vi "measure_j-v.vi"(4 "Skip pixel?":bool, 5 "Date array":string[](array[string]), 6 "Scan settings":T1={"J-V scan"=TRUE, "J-t scan"=FALSE, "Min voltage (V)"=0.0, "Max voltage (V)"=1.4, "Step (V)"=0.01, "Measurement delay (ms)"=10.0, "1st scan FB-SC"=TRUE, "Inverted structure"=FALSE, "Stabilisation time (s)"=0.0, "Stabilisation mode"=0, "Stabilisation value (V or A) "=0.0, "Step time (s)"=1.0, "Integration time"=0, "Repeat light scans"=FALSE, "Stabilisation in the dark?"=FALSE, "J-t Min (V)"=0.0, "J-t Max (V)"=1.4, "J-t Step (V)"=0.01, "Max. power stabilisation"=FALSE, "J-t 1st scan FB-SC"=TRUE, "J-t Inverted structure"=FALSE, "Max power tracking"=FALSE, "Vmp (V)"=0.7, "Total stabilisation time (s)"=100.0, "J-t best pixel only"=0, "Max power best pixel only"=0, "Vmp from J-V scan"=FALSE, "No. of repeat scans"=2.0, "Only repeat for best pixel"=0, "Stabilisation time step (s)"=1.0, "Illumination conditions"=2, "Scan rate min (V/s)"=0.1, "Scan rate max (V/s)"=1.0, "No. of scan rate steps"=1.0, "Scan rate voltage step priority"=FALSE, "Scan rate measurement delay priority"=FALSE, "J-t Illumination conditions"=0, "Max P stab. Specific voltage"=FALSE} {"J-t Illumination conditions" items=["Light only", "Dark only", "Light then dark", "Dark then light"]; "No. of scan rate steps" min=1.0 step=1.0; "Illumination conditions" items=["Light only", "Dark only", "Light then dark", "Dark then light", "Light then dark then light", "Dark then light then dark"]; "Only repeat for best pixel" items=["only for best pixel", "for best 2 pixels", "for best 3 pixels", "for best 4 pixels", "for best 5 pixels", "for best 6 pixels", "for best 7 pixels", "for all pixels"]; "No. of repeat scans" min=1.0 step=1.0; "Max power best pixel only" items=["only the best pixel", "the best 2 pixels", "the best 3 pixels", "the best 4 pixels", "the best 5 pixels", "the best 6 pixels", "the best 7 pixels", "all pixels"]; "J-t best pixel only" items=["only the best pixel", "the best 2 pixels", "the best 3 pixels", "the best 4 pixels", "the best 5 pixels", "the best 6 pixels", "the best 7 pixels", "all pixels"]; "Integration time" items=["Fast", "Normal", "High Accuracy"]; "Stabilisation mode" items=["V", "I"]; "Measurement delay (ms)" min=10.0}, 7 "Cell details cluster":T3={"Cell Position"=16, "Cell Label"="", "Pixel to measure"=0, "Area (cm^2)"=0.126, "Variable"="", "Variable value"="", "Scan settings in queue"=0, "Light or dark"="", "Measurement type"=""} {"Pixel to measure" items=["All", "1", "2", "3", "4", "5", "6", "7", "8"]}, 8 "Intensity (no. of suns)":string, 9 "Scan rate (V/s)":dbl, 10 "Experiment Title":string, 11 "User Name":string) -> (0 "Log Table":string[][](table), 2 "File path for master log":path, 3 "JV Curve":cluster{"Y":dbl[], "Y":dbl[]}[](graph))   [LabVIEW 2016]
uses:
  TypeDefs/scan_settings.ctl
  TypeDefs/Settings Boolean.ctl
  TypeDefs/nplc_for_j-v_scan.ctl
  <instrlib>/Keithley 24XX/Public/Data/Read (Single Point).vi
  <instrlib>/Keithley 24XX/Keithley 24XX.lvlib
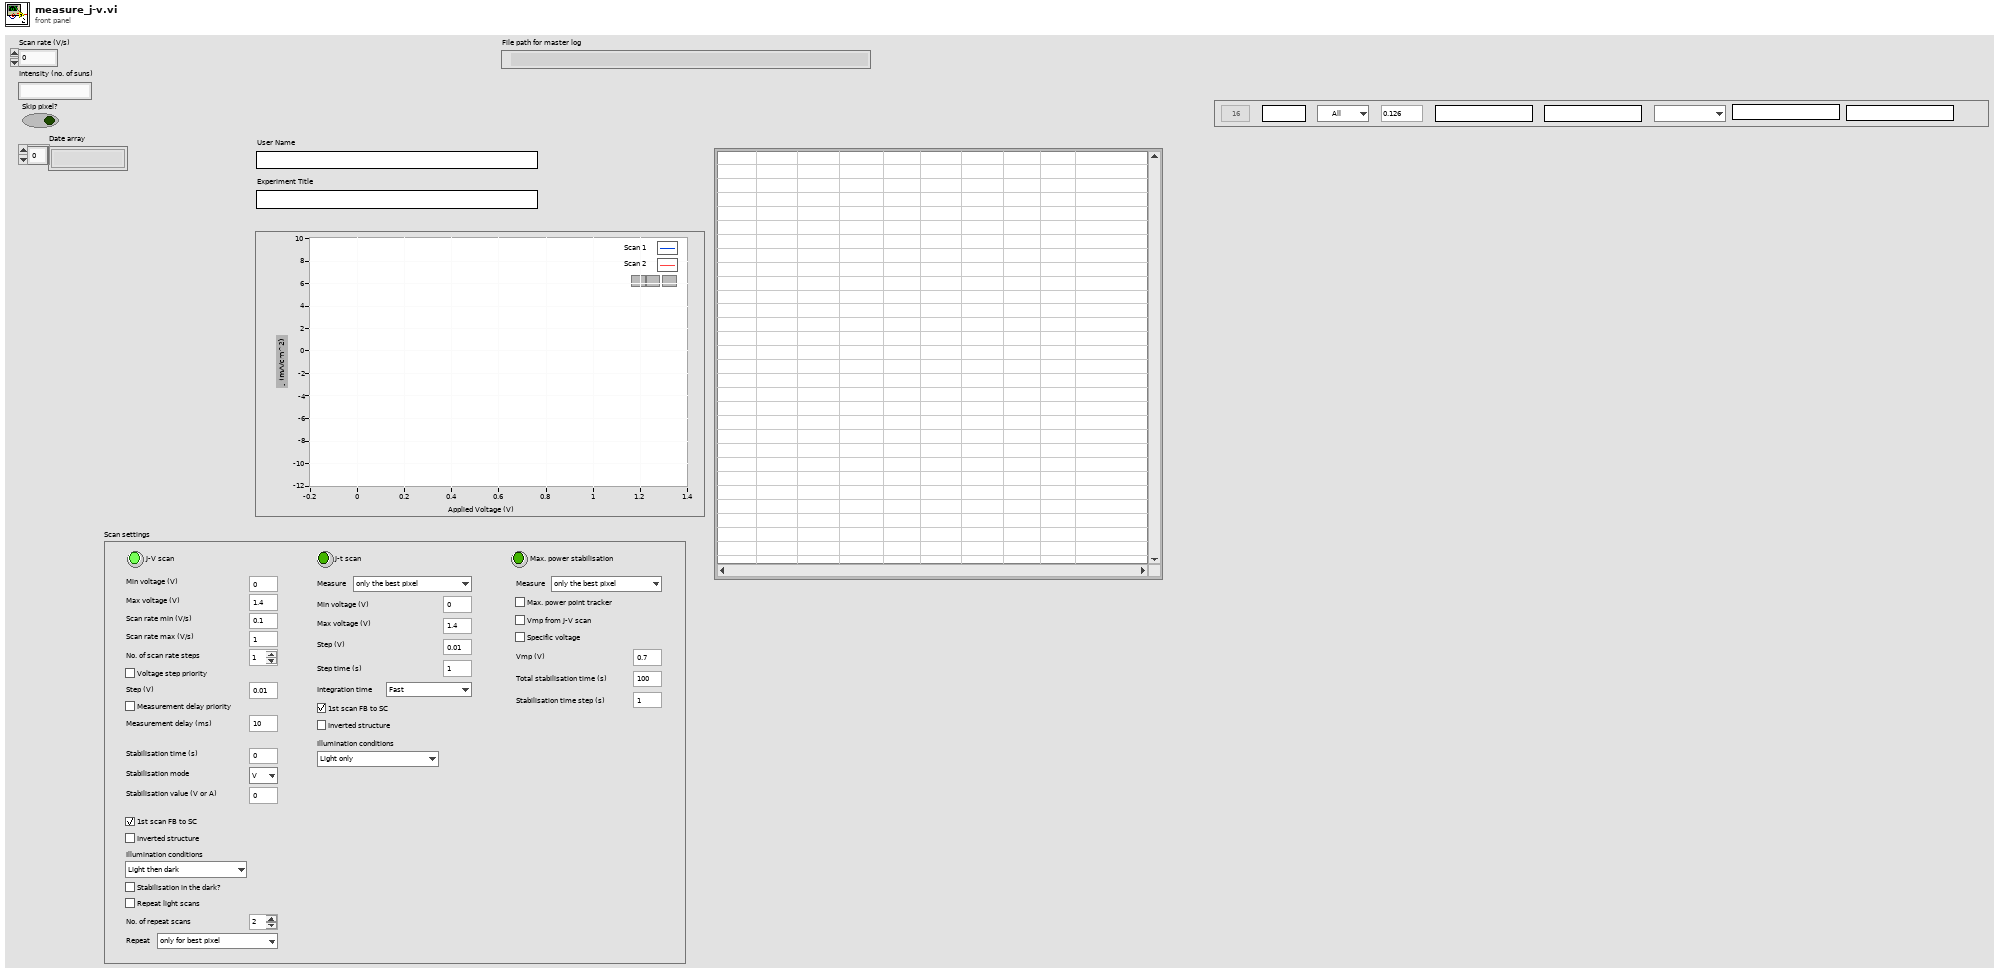
[diagram p1: front panel]
types:
  T1 = typedef "scan_settings.ctl" = cluster{"J-V scan":T2, "J-t scan":bool, "Min voltage (V)":dbl, "Max voltage (V)":dbl, "Step (V)":dbl, "Measurement delay (ms)":dbl, "1st scan FB-SC":bool, "Inverted structure":bool, "Stabilisation time (s)":dbl, "Stabilisation mode":u16, "Stabilisation value (V or A) ":dbl, "Step time (s)":dbl, "Integration time":u16, "Repeat light scans":bool, "Stabilisation in the dark?":bool, "J-t Min (V)":dbl, "J-t Max (V)":dbl, "J-t Step (V)":dbl, "Max. power stabilisation":bool, "J-t 1st scan FB-SC":bool, "J-t Inverted structure":bool, "Max power tracking":bool, "Vmp (V)":dbl, "Total stabilisation time (s)":dbl, "J-t best pixel only":u16, "Max power best pixel only":u16, "Vmp from J-V scan":bool, "No. of repeat scans":dbl, "Only repeat for best pixel":u16, "Stabilisation time step (s)":dbl, "Illumination conditions":u16, "Scan rate min (V/s)":dbl, "Scan rate max (V/s)":dbl, "No. of scan rate steps":dbl, "Scan rate voltage step priority":bool, "Scan rate measurement delay priority":bool, "J-t Illumination conditions":u16, "Max P stab. Specific voltage":bool}
  T2 = typedef "Settings Boolean.ctl" = bool
  T3 = cluster{"Cell Position":i32, "Cell Label":string, "Pixel to measure":u16, "Area (cm^2)":dbl, "Variable":string, "Variable value":string, "Scan settings in queue":u16, "Light or dark":string, "Measurement type":string}
  T4 = typedef "nplc_for_j-v_scan.ctl" = dbl
  T5 = typedef "imagedata.ctl" = cluster{"image type":i32, "image depth":i32, "image":u8[], "mask":u8[], "colors":u32[], "Rectangle":cluster{"left":i16, "top":i16, "right":i16, "bottom":i16}}
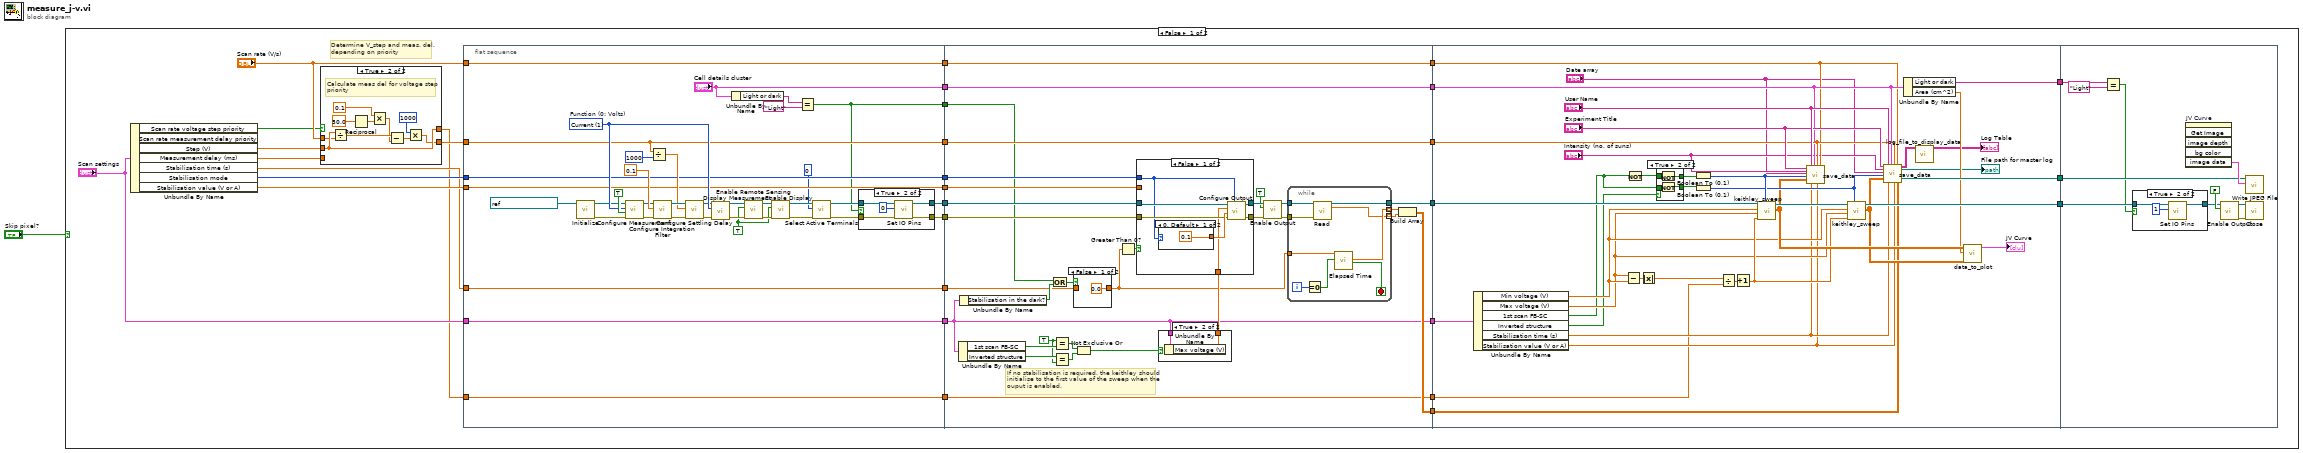
[diagram p0: block diagram]
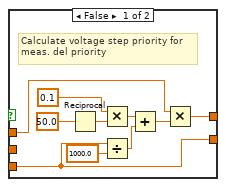
[diagram p2: hidden frame]
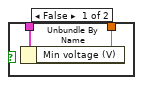
[diagram p5: hidden frame]
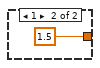
[diagram p6: hidden frame]
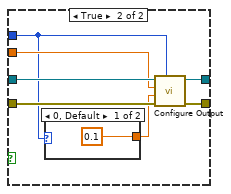
[diagram p7: hidden frame]
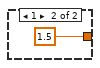
[diagram p8: hidden frame]
diagram:
  n1 = case shown="False" "Skip pixel?" {
    frame False {
      # "Determine V_step and meas. del.\ndepending on priority"
      n2 = Unbundle By Name("Scan settings") -> ("Scan rate voltage step priority"=w2:bool, "Step (V)"=w4:dbl, "Measurement delay (ms)"=w6:dbl, "Stabilisation time (s)"=w8:dbl, "Stabilisation mode"=w10:u16, "Stabilisation value (V or A)"=w11:dbl)  [unwired: 1 out]
      n3 = case shown="True" w2 {
        tunnel: [w38 w46] -> w7
        tunnel: w6 -> [w38 _]
        tunnel: "Scan rate (V/s)" -> [w34 w43]
        tunnel: [w33 w52] -> w5
        tunnel: w4 -> [_ w52]
        frame False {
          # "Calculate voltage step priority for\nmeas. del priority"
          n4 = Reciprocal(x=50.0) -> (1/x=w41:dbl)
          n5 = Multiply(x=T4 0.1, y=w41) -> (x*y=w39:T4)
          n6 = Divide(x=w38, y=1000.0) -> (x/y=w36:dbl)
          n7 = Add(x=w39, y=w36) -> (x+y=w35:T4)
          n8 = Multiply(x=w34, y=w35) -> (x*y=w33:T4)
        }
        frame True {
          # "Calculate meas del for voltage step\npriority"
          n9 = Divide(x=w52, y=w43) -> (x/y=w48:dbl)
          n10 = Reciprocal(x=50.0) -> (1/x=w50:dbl)
          n11 = Multiply(x=T4 0.1, y=w50) -> (x*y=w47:T4)
          n12 = Subtract(x=w48, y=w47) -> (x-y=w45:T4)
          n13 = Multiply(x=1000, y=w45) -> (x*y=w46:T4)
        }
      }
      n14 = flat-sequence {
        tunnel: [w70] -> w32
        tunnel: [w63] -> w31
        tunnel: [w64] -> w30
        tunnel: w11 -> [w70]
        tunnel: [w69] -> w29
        tunnel: w10 -> [w69]
        tunnel: [w68] -> w28
        tunnel: w8 -> [w68]
        tunnel: w7 -> [w67]
        tunnel: [w67] -> w27
        tunnel: [w66] -> w26
        tunnel: "Scan settings" -> [w66]
        tunnel: ["Cell details cluster"] -> w25
        tunnel: [w55] -> w24
        tunnel: [w54] -> w23
        tunnel: w5 -> [w54]
        tunnel: [w53] -> w22
        tunnel: "Scan rate (V/s)" -> [w53]
        tunnel: w32 -> [w116]
        tunnel: w31 -> [w124]
        tunnel: w30 -> [w125]
        tunnel: [w120] -> w21
        tunnel: [w117] -> w20
        tunnel: w29 -> [w113]
        tunnel: w28 -> [w99]
        tunnel: [w115] -> w19
        tunnel: w27 -> [w115]
        tunnel: [w104] -> w18
        tunnel: w26 -> [w104]
        tunnel: [w114] -> w17
        tunnel: w25 -> [w114]
        tunnel: w24 -> [w102]
        tunnel: [w98] -> w16
        tunnel: w23 -> [w98]
        tunnel: [w97] -> w15
        tunnel: w22 -> [w97]
        tunnel: [w190] -> w14
        tunnel: [w183] -> w13
        tunnel: w21 -> [w197]
        tunnel: w20 -> [w182]
        tunnel: w19 -> [w179]
        tunnel: w18 -> [w178]
        tunnel: w17 -> [w172]
        tunnel: [w171] -> w12
        tunnel: w16 -> [w164]
        tunnel: w15 -> [w163]
        tunnel: w14 -> [w208]
        tunnel: w13 -> [w209]
        tunnel: w12 -> [w204]
        frame #0 {
          w71 = TRUE ("Enable Output (T: Enable)")
          w84 = u16 1 items=["Volts", "Current", "Resistance"]  # Function (0: Volts)
          n15 = call <instrlib>:"Initialize.vi"("VISA resource name"=refnum<visa-resource-name> "GPIB1::24::INSTR") -> ("error out"=w74:errorcluster, "VISA resource name out"=w75:refnum<visa-resource-name>)  [unwired: 4 in, 5 out]
          n16 = call <instrlib>:"Configure Measurement.vi"("error in (no error)"=w74, "Enable Auto Range (T:Enable)"=TRUE, "Function (0: Volts)"=w84, "VISA resource name"=w75) -> ("error out"=w77:errorcluster, "VISA resource name out"=w76:refnum<visa-resource-name>)  [unwired: 6 in]
          n17 = Divide(x=w67, y=1000) -> (x/y=w83:T4)
          n18 = call <instrlib>:"Configure Integration Filter.vi"("error in (no error)"=w77, "Measurement Speed (1 PLC)"=T4 0.1, "VISA resource name"=w76) -> ("error out"=w86:errorcluster, "VISA resource name out"=w85:refnum<visa-resource-name>)  [unwired: 7 in]
          n19 = call <instrlib>:"Configure Settling Delay.vi"("error in (no error)"=w86, "Manual Settling Delay (0 sec)"=w83, "VISA resource name"=w85) -> ("error out"=w81:errorcluster, "VISA resource name out"=w80:refnum<visa-resource-name>)  [unwired: 7 in]
          n20 = call <instrlib>:"Display Measurement.vi"("error in (no error)"=w81, "Displayed Measurement (0: Voltage)"=w84, "VISA resource name"=w80) -> ("error out"=w79:errorcluster, "VISA resource name out"=w78:refnum<visa-resource-name>)  [unwired: 7 in]
          n21 = Unbundle By Name("Cell details cluster") -> ("Light or dark"=w62:string)
          n22 = call <instrlib>:"Enable Remote Sensing.vi"("error in (no error)"=w79, "Enable Remote Sensing (T: Enable)"=w71, "VISA resource name"=w78) -> ("error out"=w72:errorcluster, "VISA resource name out"=w73:refnum<visa-resource-name>)  [unwired: 7 in]
          n23 = call <instrlib>:"Enable Display.vi"("error in (no error)"=w72, "Enable Display (T: Enable)"=w71, "VISA resource name"=w73) -> ("error out"=w59:errorcluster, "VISA resource name out"=w60:refnum<visa-resource-name>)  [unwired: 7 in]
          n24 = Equal?(x=w62, y="Light") -> (x = y?=w55:bool)
          n25 = call <instrlib>:"Select Active Terminals.vi"("error in (no error)"=w59, "Active Terminals (0: Front)"=0, "VISA resource name"=w60) -> ("error out"=w57:errorcluster, "VISA resource name out"=w58:refnum<visa-resource-name>)  [unwired: 7 in]
          n26 = case shown="True" w55 {
            tunnel: w58 -> [w91 w95]
            tunnel: w57 -> [w90 w94]
            tunnel: [w91 w93] -> w64
            tunnel: [w90 w92] -> w63
            frame False {
            }
            frame True {
              n27 = call <instrlib>:"Set IO Pins.vi"("error in (no error)"=w94, "Output Pattern (0)"=0, "VISA resource name"=w95) -> ("error out"=w92:errorcluster, "VISA resource name out"=w93:refnum<visa-resource-name>)  [unwired: 7 in]
            }
          }
        }
        frame #1 {
          w109 = TRUE
          # "If no stabilisation is required, the keithley should\ninitialise to the first value of the sweep when the\nouput is enabled."
          n28 = Unbundle By Name(w104) -> ("1st scan FB-SC"=w111:bool, "Inverted structure"=w110:bool)
          n29 = Unbundle By Name(w104) -> ("Stabilisation in the dark?"=w103:bool)
          n30 = Or(x=w102, y=w103) -> (x .or. y?=w101:bool)
          n31 = Equal?(x=w109, y=w111) -> (x = y?=w107:bool)
          n32 = Equal?(x=w110, y=w109) -> (x = y?=w106:bool)
          n33 = case shown="False" w101 {
            tunnel: [0.0 ("Stabilisation time (s)") w129] -> w100
            tunnel: w99 -> [_ w129]
            frame False {
            }
            frame True {
            }
          }
          n34 = Not Exclusive Or(1:w106, 2:w107) -> (0:w105:bool)
          n35 = Greater Than 0?(x=w100) -> (x > 0?=w112:bool)
          n36 = case shown="True" w105 {
            tunnel: w104 -> [w130 w133]
            tunnel: [w131 w132] -> w108
            frame False {
              n37 = Unbundle By Name(w130) -> ("Min voltage (V)"=w131:dbl)
            }
            frame True {
              n38 = Unbundle By Name(w133) -> ("Max voltage (V)"=w132:dbl)
            }
          }
          n39 = case shown="False" w112 {
            tunnel: [w138 w149] -> w127
            tunnel: [w139 w148] -> w126
            tunnel: w125 -> [w136 w147]
            tunnel: w124 -> [w137 w146]
            tunnel: w116 -> [_ w145]
            tunnel: w113 -> [w135 w144]
            tunnel: w108 -> [w134 _]
            frame False {
              n40 = case shown="0, Default" w135 {
                tunnel: [0.1 1.5] -> w140
                frame 0, Default {
                }
                frame 1 {
                }
              }
              n41 = call <instrlib>:"Configure Output.vi"("Source Mode  (0: Voltage)"=w135, "error in (no error)"=w137, "Compliance  Level (0.1)"=w140, "Output Level (0)"=w134, "VISA resource name"=w136) -> ("error out"=w138:errorcluster, "VISA resource name out"=w139:refnum<visa-resource-name>)  [unwired: 5 in]
            }
            frame True {
              n42 = case shown="0, Default" w144 {
                tunnel: [0.1 1.5] -> w143
                frame 0, Default {
                }
                frame 1 {
                }
              }
              n43 = call <instrlib>:"Configure Output.vi"("Source Mode  (0: Voltage)"=w144, "error in (no error)"=w146, "Compliance  Level (0.1)"=w143, "Output Level (0)"=w145, "VISA resource name"=w147) -> ("error out"=w149:errorcluster, "VISA resource name out"=w148:refnum<visa-resource-name>)  [unwired: 5 in]
            }
          }
          n44 = call <instrlib>:"Enable Output.vi"("error in (no error)"=w127, "Enable Output (T: Enable)"=TRUE ("Output (Off)"), "VISA resource name"=w126) -> ("error out"=w121:errorcluster, "VISA resource name out"=w122:refnum<visa-resource-name>)  [unwired: 7 in]
          n45 = while {
            tunnel: w122 -> [w160]
            tunnel: w121 -> [w159]
            tunnel: [w158] -> w120
            tunnel: [w156] -> w119 mode=indexing
            tunnel: [w155] -> w118 mode=indexing
            tunnel: w100 -> [w152]
            i -> [w154]
            stop <- w157 stop-if-true
            n46 = Equal To 0?(x=w154) -> (x = 0?=w153:bool)
            n47 = call-poly <instrlib>:"Read.vi"("VISA resource name"=w160, "error in (no error)"=w159) -> ("VISA resource name out"=w158:refnum<visa-resource-name>, "Current"=w155:sgl)  [unwired: 7 in, 5 out]
            n48 = call "Elapsed Time"("Time Target (s)"=w152, "Reset"=w153) -> ("Elapsed Time (s)"=w156:dbl, "Time has Elapsed"=w157:bool)  [unwired: 10 in, 6 out]
          }
          n49 = Build Array(w119, w118) -> (w117:dbl[][])
        }
        frame #2 {
          n50 = Unbundle By Name(w178) -> ("Min voltage (V)"=w177:dbl, "Max voltage (V)"=w176:dbl, "1st scan FB-SC"=w166:bool, "Inverted structure"=w175:bool, "Stabilisation time (s)"=w174:dbl, "Stabilisation value (V or A)"=w173:dbl)
          n51 = Subtract(x=w176, y=w177) -> (x-y=w195:dbl)
          n52 = Not(x=w166) -> (.not. x?=w167:bool)
          n53 = Absolute Value(x=w195) -> (abs(x)=w196:dbl)
          n54 = case shown="True" w175 {
            tunnel: [w199 w203] -> w185
            tunnel: [w198 w202] -> w184
            tunnel: w166 -> [w198 w201]
            tunnel: w167 -> [w199 w200]
            frame False {
            }
            frame True {
              n55 = Not(x=w200) -> (.not. x?=w203:bool)
              n56 = Not(x=w201) -> (.not. x?=w202:bool)
            }
          }
          n57 = Boolean To (0,1)(Boolean=w185) -> (0, 1=w193:i16)
          n58 = Boolean To (0,1)(Boolean=w184) -> (0, 1=w191:i16)
          n59 = Divide(x=w196, y=w164) -> (x/y=w187:T4)
          n60 = Increment(x=w187) -> (x+1=w186:T4)
          n61 = call "keithley_sweep.vi"("Sweep Direction"=w193, "Number of Points"=w186, "Maximum Amplitude"=w176, "Minimum Amplitude"=w177, "VISA resource name out 2"=w197) -> ("Data Array"=w189:dbl[][], "VISA resource name out"=w192:refnum<visa-resource-name>)  [unwired: 2 in, 1 out]
          n62 = call "save_data.vi"("Experiment Indicator"="Experiment Title", "Intensity (no. of suns)"="Intensity (no. of suns)", "Date array"="Date array", "Scan direction"=w193, "Data Array"=w189, "Username"="User Name", "Stabilisation time (ms)"=w174, "Cell details cluster"=w172, "Measurement Delay (ms)"=w179, "Stabilisation level \n(A or V depending on mode)"=w173, "Scan rate (V/s)"=w163) -> ()  [unwired: 5 in, 4 out]
          n63 = call "keithley_sweep.vi"("Sweep Direction"=w191, "Number of Points"=w186, "Maximum Amplitude"=w176, "Minimum Amplitude"=w177, "VISA resource name out 2"=w192) -> ("Data Array"=w188:dbl[][], "VISA resource name out"=w190:refnum<visa-resource-name>)  [unwired: 2 in, 1 out]
          n64 = call "save_data.vi"("Experiment Indicator"="Experiment Title", "Intensity (no. of suns)"="Intensity (no. of suns)", "Date array"="Date array", "Scan direction"=w191, "Data Array"=w188, "Username"="User Name", "Stabilisation time (ms)"=w174, "Cell details cluster"=w172, "Measurement Delay (ms)"=w179, "Stabilisation level \n(A or V depending on mode)"=w173, "Scan rate (V/s)"=w163, "Stabilisation Data"=w182) -> ("Master Log"=w169:string[][], "File path for master log"=→"File path for master log":path, "File path for JV image"=w183:path)  [unwired: 4 in, 1 out]
          n65 = Unbundle By Name(w172) -> ("Light or dark"=w171:string, "Area (cm^2)"=w170:dbl)
          n66 = call "log_file_to_display_data.vi"("Master Log"=w169) -> ("Formatted table"=→"Log Table":string[][])  [unwired: 10 in]
          n67 = call "data_to_plot.vi"("Data Array 2"=w188, "Device Area (cm^2)"=w170, "Data Array"=w189) -> ("JV Curve"=→"JV Curve":cluster{"Y":dbl[], "Y":dbl[]}[])  [unwired: 8 in]
        }
        frame #3 {
          n68 = Equal?(x=w204, y="Light") -> (x = y?=w205:bool)
          n69 = case shown="True" w205 {
            tunnel: w208 -> [w214 w216]
            tunnel: [w214 w215] -> w207
            frame False {
            }
            frame True {
              n70 = call <instrlib>:"Set IO Pins.vi"("Output Pattern (0)"=1, "VISA resource name"=w216) -> ("VISA resource name out"=w215:refnum<visa-resource-name>)  [unwired: 8 in, 1 out]
            }
          }
          n71 = invoke on="JV Curve" class="XYGraph (strict)" method="Get Image"() -> ("image data"=w210:T5)  [unwired: 6 in, 5 out]
          n72 = call <instrlib>:"Enable Output.vi"("Enable Output (T: Enable)"=FALSE ("Output (Off)"), "VISA resource name"=w207) -> ("error out"=w212:errorcluster, "VISA resource name out"=w213:refnum<visa-resource-name>)  [unwired: 8 in]
          n73 = call <vilib>:"Write JPEG File.vi"("image data"=w210, "path to JPEG file"=w209) -> ()  [unwired: 8 in, 2 out]
          n74 = call <instrlib>:"Close.vi"("error in (no error)"=w212, "VISA resource name"=w213) -> ()  [unwired: 9 in, 1 out]
        }
      }
    }
    frame True {
    }
  }
